vi "SDO_SIM_SIM_INIT.vi"(8 "error in (no error)":errorcluster, 11 "Initial Robot Position":T1 {"ROTATION"."SIN" format="%13.4f"; "ROTATION"."COS" format="%13.4f"; "ROTATION"."VALUE" format="%13.4f"; "TRANSLATION"."Y" format="%14.3f"; "TRANSLATION"."X" format="%14.3f"}) -> (0 "error out":errorcluster)   [LabVIEW 2019]
uses:
  <vilib>/Rock Robotics/WPI/ThirdParty/JAS_Junk/TrajLib/TypeDef/POSE2D.ctl
  <vilib>/Rock Robotics/WPI/ThirdParty/JAS_Junk/TrajLib/TypeDef/TRANSLATION2D.ctl
  <vilib>/Rock Robotics/WPI/ThirdParty/JAS_Junk/TrajLib/TypeDef/ROTATION2D.ctl
  <vilib>/Rock Robotics/SystemInterfaces/DIO/FPGA_DIOPWMChannel.ctl
  <vilib>/Rock Robotics/SystemInterfaces/DIO/FPGA_DIOChannel.ctl
  <vilib>/Rock Robotics/WPI/ThirdParty/JAS_Junk/TrajLib/Conv_Deg_Radians.vi
  <vilib>/Rock Robotics/WPI/ThirdParty/JAS_Junk/TrajLib/Rotation2d_CreateAngle.vi
  SDO_SIM_SIM_Globals.vi
  <vilib>/Rock Robotics/WPI/ThirdParty/JAS_Junk/TrajLib/Trajectory_Library.lvlib
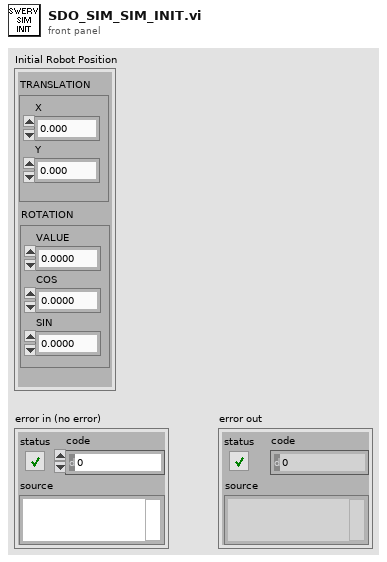
[diagram p1: front panel]
types:
  T1 = typedef "Trajectory_Library.lvlib/POSE2D.ctl" = cluster{"TRANSLATION":T2, "ROTATION":T3}
  T2 = typedef "Trajectory_Library.lvlib/TRANSLATION2D.ctl" = cluster{"X":dbl, "Y":dbl}
  T3 = typedef "Trajectory_Library.lvlib/ROTATION2D.ctl" = cluster{"VALUE":dbl, "COS":dbl, "SIN":dbl}
  T4 = typedef "FPGA_DIOChannel.ctl" = enum8{"DIO 0", "DIO 1", "DIO 2", "DIO 3", "DIO 4", "DIO 5", "DIO 6", "DIO 7", "DIO 8", "DIO 9", "DIO MXP 0", "DIO MXP 1", "DIO MXP 2", "DIO MXP 3", "DIO MXP 4", "DIO MXP 5", "DIO MXP 6", "DIO MXP 7", "DIO MXP 8", "DIO MXP 9", "DIO MXP 10", "DIO MXP 11", "DIO MXP 12", "DIO MXP 13", "DIO MXP 14", "DIO MXP 15", "SPI Port CS1", "SPI Port CS2", "SPI Port CS3", "SPI Port MISO", "SPI Port MOSI", "Invalid"}
  T5 = typedef "FPGA_DIOPWMChannel.ctl" = enum8{"PWM 0", "PWM 1", "PWM 2", "PWM 3", "PWM 4", "PWM 5", "PWM 6", "PWM 7", "PWM 8", "PWM 9", "PWM MXP 0", "PWM MXP 1", "PWM MXP 2", "PWM MXP 3", "PWM MXP 4", "PWM MXP 5", "PWM MXP 6", "PWM MXP 7", "PWM MXP 8", "PWM MXP 9", "Invalid"}
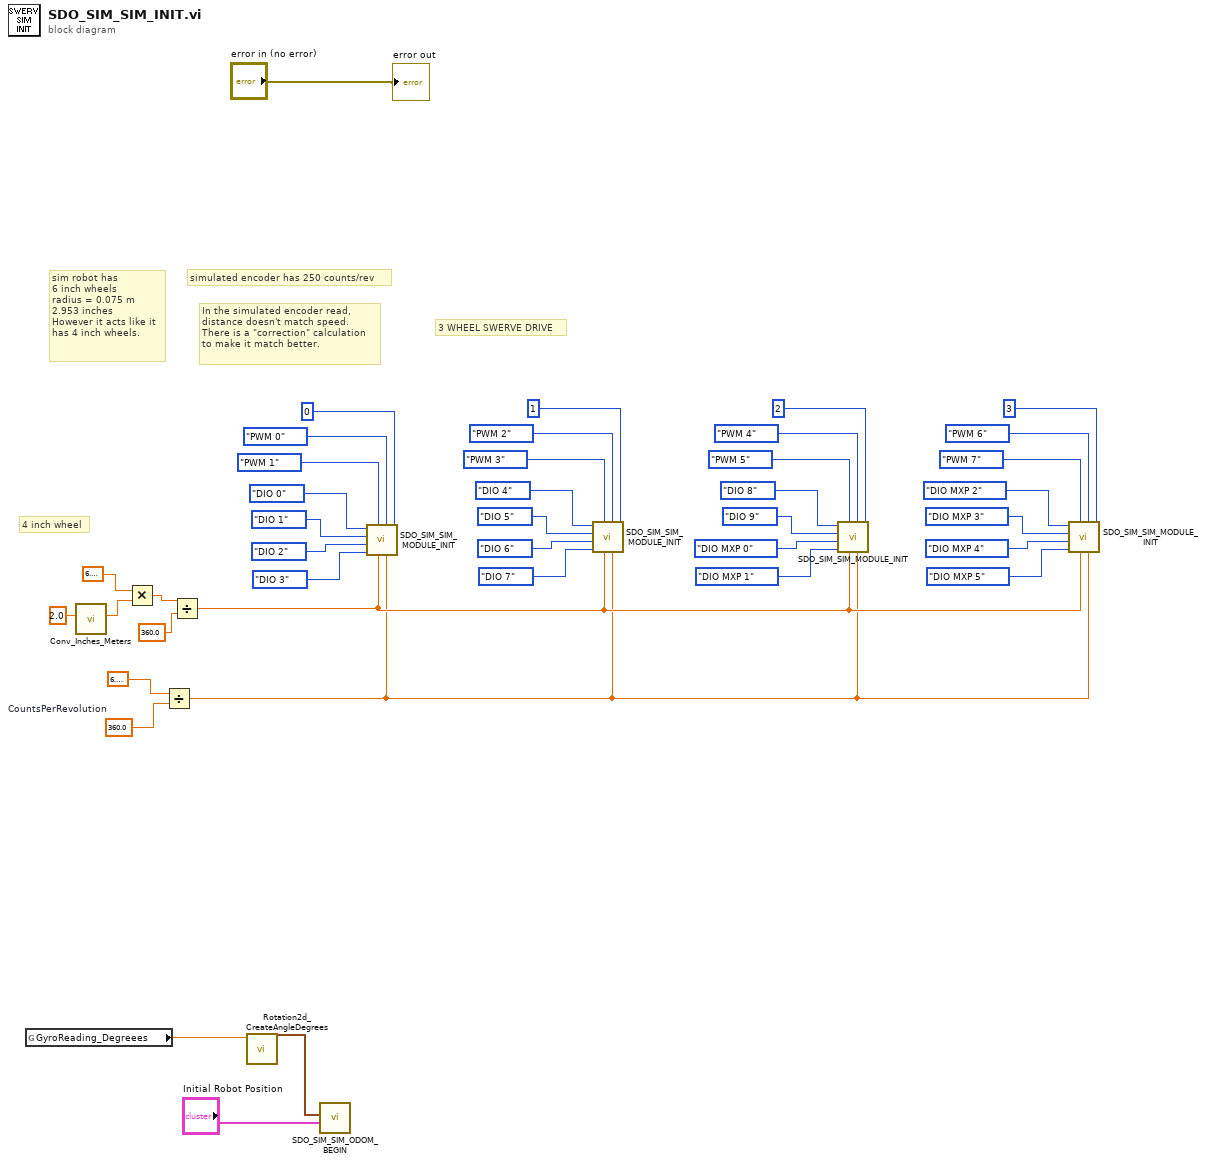
[diagram p0: block diagram]
diagram:
  w16 = 360.0  # CountsPerRevolution
  # "4 inch wheel"
  # "3 WHEEL SWERVE DRIVE"
  # "In the simulated encoder read,\ndistance doesn't match speed.\nThere is a \"correction\" calculation\nto make it match better."
  # "simulated encoder has 250 counts/rev"
  # "sim robot has\n6 inch wheels\nradius = 0.075 m\n2.953 inches\nHowever it acts like it\nhas 4 inch wheels."
  n1 = global read "SDO_SIM_SIM_Globals.vi" "GyroReading_Degreees"() -> (w2:dbl)
  n2 = call <vilib>:"Conv_Inches_Meters.vi"("INCH"=2.0) -> ("Meters"=w31:dbl)  [unwired: 10 in]
  n3 = Multiply(x=6.283185307179586, y=w31) -> (x*y=w5:dbl)
  n4 = Divide(x=6.283185307179586, y=w16) -> (x/y=w40:dbl)
  n5 = Divide(x=w5, y=360.0) -> (x/y=w41:dbl)
  n6 = call <vilib>:"Rotation2d_CreateAngleDegrees.vi"("Angle_Degrees"=w2) -> ("ROTATION"=w1:T3)  [unwired: 10 in]
  n7 = call "SDO_SIM_SIM_ODOM_BEGIN.vi"("Initial Pose"="Initial Robot Position", "Initial Gyro Angle"=w1) -> ()  [unwired: 9 in, 1 out]
  n8 = call "SDO_SIM_SIM_MODULE_INIT.vi"("Module Index"=0 ("NameSuffix"), "SwerveRadiansPerCount"=w40, "Drive PWM Channel"=FPGA_DIOPWMChannel."PWM 0", "DriveDistPerCount"=w41, "Swerve PWM Channel"=FPGA_DIOPWMChannel."PWM 1", "Swerve B Channel"=FPGA_DIOChannel."DIO 3", "Swerver A Channel"=FPGA_DIOChannel."DIO 2", "Drive B Channel"=FPGA_DIOChannel."DIO 1", "Drive A channel"=FPGA_DIOChannel."DIO 0") -> ()  [unwired: 3 in]
  n9 = call "SDO_SIM_SIM_MODULE_INIT.vi"("Module Index"=1 ("NameSuffix"), "SwerveRadiansPerCount"=w40, "Drive PWM Channel"=FPGA_DIOPWMChannel."PWM 2", "DriveDistPerCount"=w41, "Swerve PWM Channel"=FPGA_DIOPWMChannel."PWM 3", "Swerve B Channel"=FPGA_DIOChannel."DIO 7", "Swerver A Channel"=FPGA_DIOChannel."DIO 6", "Drive B Channel"=FPGA_DIOChannel."DIO 5", "Drive A channel"=FPGA_DIOChannel."DIO 4") -> ()  [unwired: 3 in]
  n10 = call "SDO_SIM_SIM_MODULE_INIT.vi"("Module Index"=2 ("NameSuffix"), "SwerveRadiansPerCount"=w40, "Drive PWM Channel"=FPGA_DIOPWMChannel."PWM 4", "DriveDistPerCount"=w41, "Swerve PWM Channel"=FPGA_DIOPWMChannel."PWM 5", "Swerve B Channel"=FPGA_DIOChannel."DIO MXP 1", "Swerver A Channel"=FPGA_DIOChannel."DIO MXP 0", "Drive B Channel"=FPGA_DIOChannel."DIO 9", "Drive A channel"=FPGA_DIOChannel."DIO 8") -> ()  [unwired: 3 in]
  n11 = call "SDO_SIM_SIM_MODULE_INIT.vi"("Module Index"=3 ("NameSuffix"), "SwerveRadiansPerCount"=w40, "Drive PWM Channel"=FPGA_DIOPWMChannel."PWM 6", "DriveDistPerCount"=w41, "Swerve PWM Channel"=FPGA_DIOPWMChannel."PWM 7", "Swerve B Channel"=FPGA_DIOChannel."DIO MXP 5", "Swerver A Channel"=FPGA_DIOChannel."DIO MXP 4", "Drive B Channel"=FPGA_DIOChannel."DIO MXP 3", "Drive A channel"=FPGA_DIOChannel."DIO MXP 2") -> ()  [unwired: 3 in]
  "error out" <- "error in (no error)"
